vi "Phase difference 2010.vi"(1 "Signals":waveform(dbl)[](array[waveform]), 3 "Error In":errorcluster) -> (7 "Phase Array":dbl[](array[numeric]), 8 "Max Phase Difference":dbl, 9 "Frequency Array":dbl[](array[numeric]), 10 "Error Out":errorcluster)   [LabVIEW 2011]
doc: "This VI will find the frequency and phase difference between an array of waveforms, and can be used to test your system's\nsynchronization.\n\n1.) Performs windowing using a Hanning window on your signal to get the correct frequency components.\n2.) Obtains the Phase and Frequency Information of your waveform signal.\n3.) Find the normalized frequeny components\n4.) Outputs the various phase values, frequency values, and max phase difference"
uses:
  <vilib>/Analysis/4window.llb/Hanning Window (DBL).vi
  <vilib>/measure/matone.llb/Extract Single Tone Information 1 Chan.vi
  <vilib>/measure/NI_MAPro.lvlib
  <vilib>/Analysis/NI_AALPro.lvlib
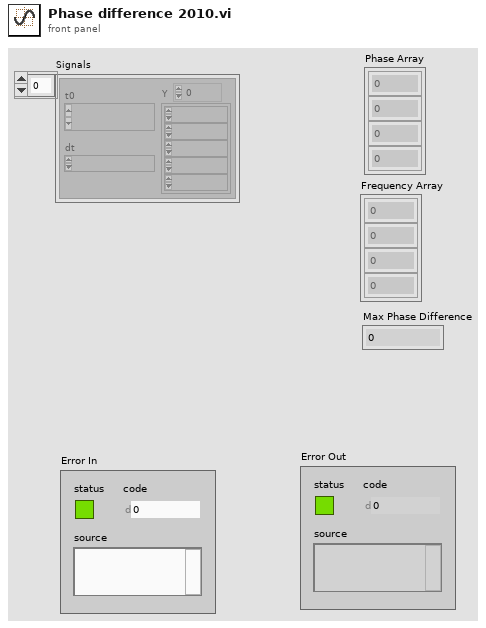
[diagram p1: front panel]
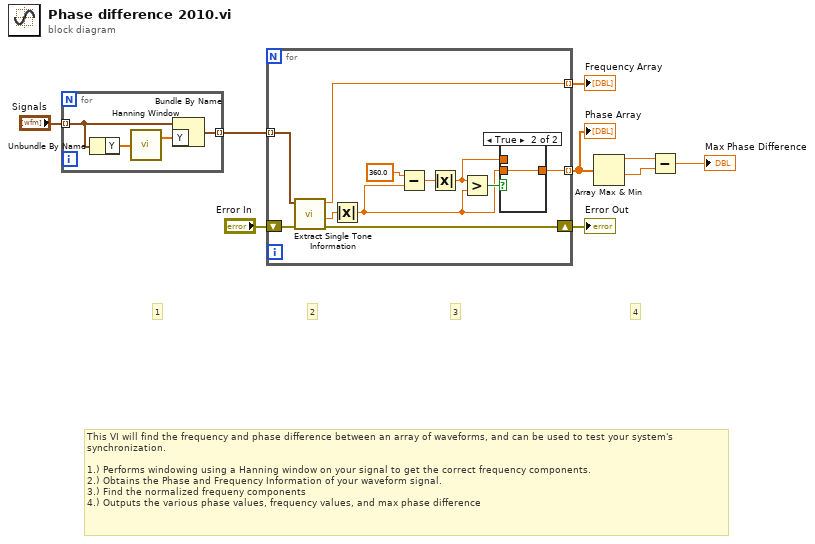
[diagram p0: block diagram]
diagram:
  # "This VI will find the frequency and phase difference between an array of waveforms, and can be used to test your system's\nsynchronization.\n\n1.) Performs windowing using a Hanning window on your signal to get the correct frequency components.\n2.) Obtains the Phase and Frequency Information of your waveform signal.\n3.) Find the normalized frequeny components\n4.) Outputs the various phase values, frequency values, and max phase difference"
  # "4"
  # "1"
  # "2"
  # "3"
  n1 = for {
    tunnel: "Signals" -> [w11] mode=indexing
    tunnel: [w10] -> w2 mode=indexing
    n2 = Unbundle By Name(w11) -> ("Y"=w12:dbl[])
    n3 = call-poly <vilib>:"Hanning Window.vi"("X"=w12) -> ("Windowed X"=w13:dbl[])  [unwired: 1 out]
    n4 = Bundle By Name(cluster=w11, "Y"=w13) -> (w10:waveform(dbl))
  }
  n5 = for {
    tunnel: w2 -> [w18] mode=indexing
    tunnel: [w17] -> w7 mode=indexing
    tunnel: [w16] -> w5 mode=indexing
    shift-right: [w14] -> w4
    shift-left: "Error In" -> [w15]
    n6 = call-poly <vilib>:"Extract Single Tone Information.vi"("error in (no error)"=w15, "time signal in"=w18) -> ("error out"=w14:errorcluster, "detected phase (deg)"=w24:dbl, "detected frequency"=w16:dbl)  [unwired: 4 in, 3 out]
    n7 = Absolute Value(x=w24) -> (abs(x)=w19:dbl)
    n8 = Subtract(x=360.0, y=w19) -> (x-y=w22:dbl)
    n9 = Absolute Value(x=w22) -> (abs(x)=w20:dbl)
    n10 = Greater?(x=w20, y=w19) -> (0:w21:bool)
    n11 = case shown="True" w21 {
      tunnel: [w25 w26] -> w17
      tunnel: w19 -> [_ w26]
      tunnel: w20 -> [w25 _]
      frame False {
      }
      frame True {
      }
    }
  }
  "Phase Array" <- w7
  "Frequency Array" <- w5
  "Error Out" <- w4
  n12 = Array Max & Min(array=w7) -> (max value=w9:dbl, min value=w8:dbl)  [unwired: 2 out]
  n13 = Subtract(x=w9, y=w8) -> (x-y=→"Max Phase Difference":dbl)
